vi "Update ini files.vi"() -> ()   [LabVIEW 2012]
uses:
  <vilib>/Utility/sysdir.llb/System Directory Type.ctl
panel:
  out "Array":errorcluster[](array[cluster])
  out "filenames":string[](array[string])
  out "text":string
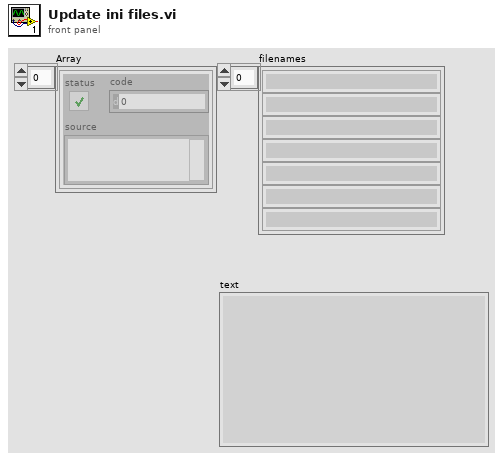
[diagram p1: front panel]
types:
  T1 = typedef "System Directory Type.ctl" = i32
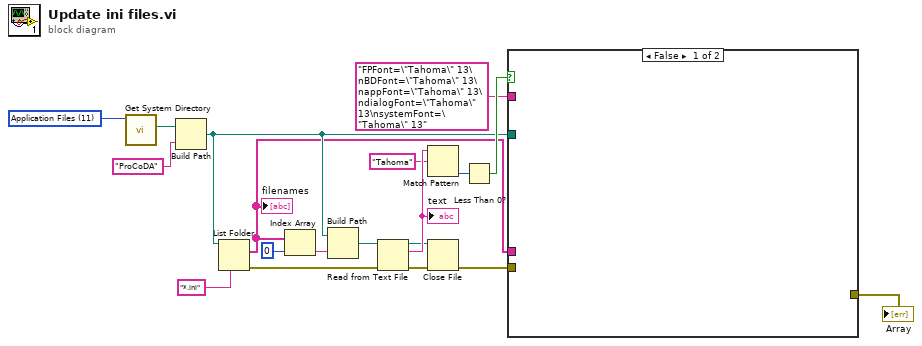
[diagram p0: block diagram]
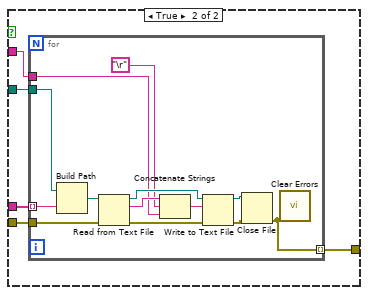
[diagram p2: hidden frame]
diagram:
  w19 = T1 11 items=["User Home"=0, "User Desktop"=1, "User Documents"=2, "User Application Data"=3, "User Preferences"=4, "User Temporary"=5, "Public Documents"=6, "Public Application Data"=7, "Public Preferences"=8, "Public Cache"=13, "System Core Libraries"=9, "System Installed Libraries"=10, "Application Files"=11, "Boot Volume Root"=12] ("system directory type")
  n1 = call <vilib>:"Get System Directory.vi"("system directory type"=w19) -> ("system directory"=w17:path)  [unwired: 10 in]
  n2 = Build Path(base path=w17, name or relative path="ProCoDA") -> (appended path=w8:path)
  n3 = List Folder(path=w8, pattern="*.ini") -> (filenames=w7:string[], error out=w2:errorcluster)  [unwired: 2 in, 2 out]
  "filenames" <- w7
  n4 = Index Array(array=w7, index=0) -> (element=w9:string)
  n5 = Build Path(base path=w8, name or relative path=w9) -> (appended path=w16:path)
  n6 = Read from Text File(file (use dialog)=w16, error in=w2) -> (refnum out=w5:refnum<file>, text=w15:string, error out=w4:errorcluster)  [unwired: 2 in, 1 out]
  "text" <- w15
  n7 = Match Pattern(string=w15, regular expression="Tahoma" ("search string")) -> (offset past match=w13:i32)  [unwired: 1 in, 3 out]
  n8 = Close File(refnum=w5, error in=w4) -> (error out=w3:errorcluster)  [unwired: 1 out]
  n9 = Less Than 0?(x=w13) -> (x < 0?=w12:bool)
  n10 = case shown="False" w12 {
    tunnel: w8 -> [_ w24]
    tunnel: w7 -> [_ w23]
    tunnel: "FPFont=\"Tahoma\" 13\nBDFont=\"Tahoma\" 13\nappFont=\"Tahoma\" 13\ndialogFont=\"Tahoma\" 13\nsystemFont=\"Tahoma\" 13" -> [_ w22]
    tunnel: w3 -> [_ w21]
    tunnel: [_ w20] -> w1
    frame False {
    }
    frame True {
      n11 = for {
        tunnel: w24 -> [w37]
        tunnel: w23 -> [w36] mode=indexing
        tunnel: w22 -> [w27]
        tunnel: w21 -> [w28]
        tunnel: [w25] -> w20 mode=indexing
        n12 = Build Path(base path=w37, name or relative path=w36) -> (appended path=w35:path)
        n13 = Read from Text File(file (use dialog)=w35, error in=w28) -> (refnum out=w30:refnum<file>, text=w34:string, error out=w29:errorcluster)  [unwired: 2 in, 1 out]
        n14 = Concatenate Strings(w34, "\r", w27) -> (w31:string)
        n15 = Write to Text File(file (use dialog)=w30, text=w31, error in=w29) -> (refnum out=w32:refnum<file>, error out=w33:errorcluster)  [unwired: 1 in, 1 out]
        n16 = Close File(refnum=w32, error in=w33) -> (error out=w25:errorcluster)  [unwired: 1 out]
        n17 = call <vilib>:"Clear Errors.vi"("error in (no error)"=w25) -> ()  [unwired: 6 in, 1 out]
      }
    }
  }
  "Array" <- w1
